vi "DriveCommandToMotorPower.vi"(8 "Drive Command Override":bool, 9 "Drive Command Override (ul) [-1,1]":dbl, 10 "Drive Command (ul) [-1,1]":dbl, 11 "Actual Shifter State":T1(ring)) -> (2 "Motor Power (ul) [-1,1]":dbl)   [LabVIEW 2019]
doc: "This VI linearizes the the drive motor behavior by converting the linear, unitless drive command to the appropriate drive motor power. Handles low and high gear shifter states. The motors shoulds be calibrated with voltage compensation switched ON."
uses:
  constants.vi
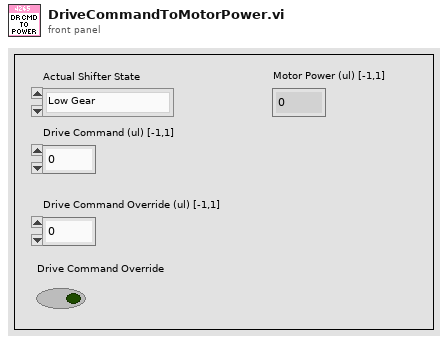
[diagram p1: front panel]
types:
  T1 = enum16{"Low Gear", "High Gear", "Transiting", "Unknown"}
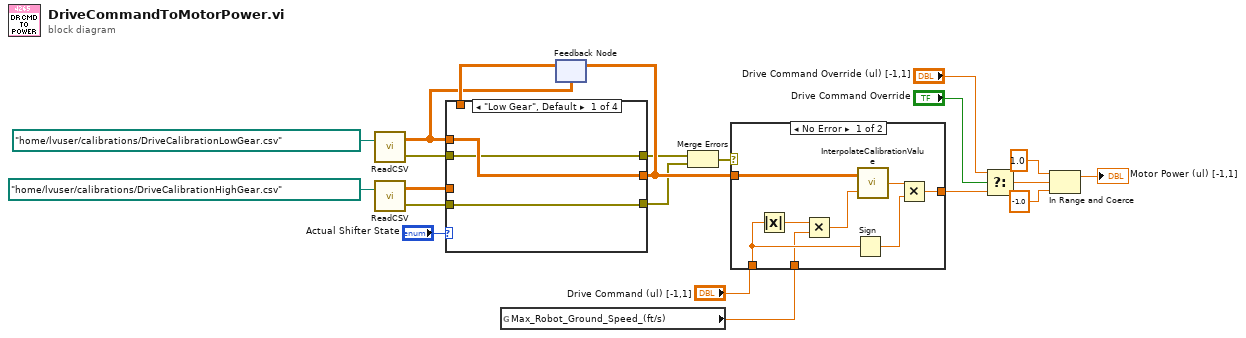
[diagram p0: block diagram]
diagram:
  n1 = call "ReadCSV.vi"("File Path (.csv)"=path "/home/lvuser/calibrations/DriveCalibrationLowGear.csv" ("path")) -> ("File Open Eror"=w14:errorcluster, "Data (index by row)"=w15:dbl[][])  [unwired: 1 in]
  n2 = call "ReadCSV.vi"("File Path (.csv)"=path "/home/lvuser/calibrations/DriveCalibrationHighGear.csv" ("path")) -> ("File Open Eror"=w12:errorcluster, "Data (index by row)"=w16:dbl[][])  [unwired: 1 in]
  n3 = global read "constants.vi" "Max_Robot_Ground_Speed_(ft/s)"() -> (w6:dbl)
  n4 = feedback #1(w15) -> (w17:dbl[][])
  n5 = case shown="\"Low Gear\", Default" "Actual Shifter State" {
    tunnel: w16 -> [_ w27 _ _]
    tunnel: w15 -> [w24 _ _ _]
    tunnel: [w24 w27 w30 w33] -> w18
    tunnel: w17 -> [_ _ w30 w33]
    tunnel: [w23 w26 w29 w32] -> w13
    tunnel: w14 -> [w23 w26 w29 w32]
    tunnel: [w22 w25 w28 w31] -> w11
    tunnel: w12 -> [w22 w25 w28 w31]
    frame "Low Gear", Default {
    }
    frame "High Gear" {
    }
    frame "Transiting" {
    }
    frame "Unknown" {
    }
  }
  n6 = feedback-in #1(w18) -> ()
  n7 = Merge Errors(w13, w11) -> (w10:errorcluster)
  n8 = case shown="No Error" w10 {
    tunnel: "Drive Command (ul) [-1,1]" -> [w39 w42]
    tunnel: [w36 w42] -> w8
    tunnel: w18 -> [w35 _]
    tunnel: w6 -> [w34 _]
    frame No Error {
      n9 = Absolute Value(x=w39) -> (abs(x)=w40:dbl)
      n10 = Multiply(x=w40, y=w34) -> (x*y=w41:dbl)
      n11 = Sign(1:w39) -> (0:w37:dbl)
      n12 = call "InterpolateCalibrationValue.vi"("Input"=w41, "Calibration Data"=w35) -> ("Interpolated Output"=w38:dbl)
      n13 = Multiply(x=w38, y=w37) -> (x*y=w36:dbl)
    }
    frame Error {
    }
  }
  n14 = Select(t="Drive Command Override (ul) [-1,1]", s="Drive Command Override", f=w8) -> (s? t:f=w4:dbl)
  n15 = In Range and Coerce(upper limit=1.0, x=w4, lower limit=-1.0) -> (coerced(x)=→"Motor Power (ul) [-1,1]":dbl)  [unwired: 1 out]
